vi "Test Generate REF Waveforms.vi"(8 "error in (no error)":errorcluster, 11 "Generator in":refnum<class "Generator.lvclass">) -> (0 "error out":errorcluster)   [LabVIEW 2019, in "Generator.lvclass"]
uses:
  Generator.lvclass
  typedefs/REF.Channel--Cluster--Array.ctl
  typedefs/Sampling--Cluster.ctl
panel:
  out "Waveform Chart":i16(graph)
  out "Intensity Graph":dbl[][](graph)
  in  "REF Channels":T1
  in  "milliseconds to wait":u32=10
  out "Updates":i32=36
  out "Waveform Graph":waveform(dbl)[](graph)
  in  "configuration.Sampling":T2
  in  "stop":bool
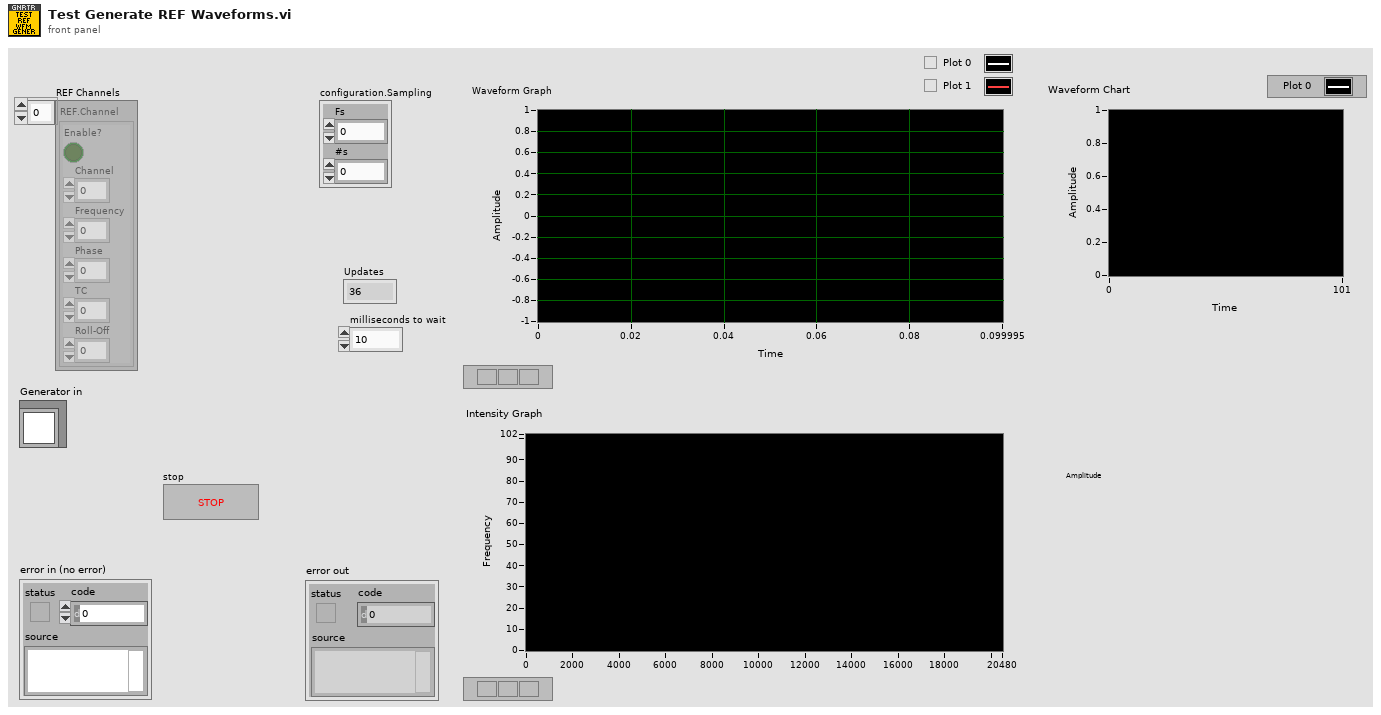
[diagram p1: front panel]
types:
  T1 = typedef "Generator.lvclass/REF.Channel--Cluster--Array.ctl" = cluster{"Enable?":bool, "Channel":i32, "Frequency":dbl, "Phase":dbl, "TC":dbl, "Roll-Off":i32}[]
  T2 = typedef "Generator.lvclass/Sampling--Cluster.ctl" = cluster{"Fs":dbl, "#s":dbl}
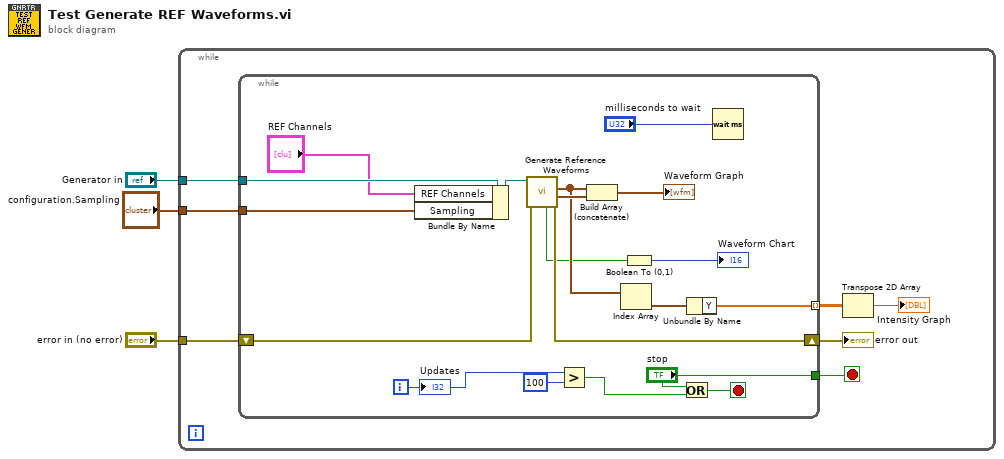
[diagram p0: block diagram]
diagram:
  n1 = while {
    tunnel: "error in (no error)" -> [w9]
    tunnel: "Generator in" -> [w6]
    tunnel: "configuration.Sampling" -> [w5]
    stop <- w4 stop-if-true
    n2 = while {
      shift-right: [w27] -> w10
      shift-left: w9 -> [w28]
      tunnel: [w19] -> w8 mode=indexing
      tunnel: w6 -> [w15]
      tunnel: w5 -> [w11]
      tunnel: ["stop"] -> w4
      i -> [w25]
      stop <- w22 stop-if-true
      n3 = Bundle By Name(cluster=w15, "REF Channels"="REF Channels", "Sampling"=w11) -> (w14:refnum<class "Generator.lvclass">)
      n4 = call "Generate Reference Waveforms.vi"("error in (no error)"=w28, "Generator in"=w14) -> ("error out"=w27:errorcluster, "REF_Y"=w26:waveform(dbl)[], "REF_X"=w21:waveform(dbl)[], "phase reset"=w17:bool)  [unwired: 5 in, 1 out]
      n5 = Greater?(x=w25, y=100) -> (0:w23:bool)
      n6 = Build Array (concatenate)(w21, w26) -> (→"Waveform Graph":waveform(dbl)[])
      n7 = Index Array(array=w21) -> (element=w20:waveform(dbl))  [unwired: 1 in]
      n8 = Boolean To (0,1)(Boolean=w17) -> (0, 1=→"Waveform Chart":i16)
      n9 = Or(x="stop", y=w23) -> (x .or. y?=w22:bool)
      n10 = Unbundle By Name(w20) -> ("Y"=w19:dbl[])
      n11 = Wait (ms)(milliseconds to wait="milliseconds to wait") -> ()  [unwired: 1 out]
      "Updates" <- w25
    }
    "error out" <- w10
    n12 = Transpose 2D Array(2D array=w8) -> (transposed array=→"Intensity Graph":dbl[][])
  }
